vi "HGF_Visitor.appendData2Variant.vi"(0 "initData":variant, 2 "addressee":string, 3 "destination":refnum<class "HGF_TriggeredEvent.lvclass">, 5 "error in (no error)":errorcluster) -> (14 "dup initData":variant, 19 "error out":errorcluster)   [LabVIEW 2014, in "HGF_BaseClasses.lvlib" / "HGF_Visitor.lvclass"]
uses:
  HGF_Visitor.lvclass
  HGF_TriggeredEvent/HGF_TriggeredEvent.lvclass
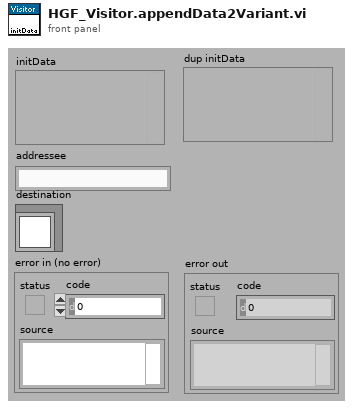
[diagram p1: front panel]
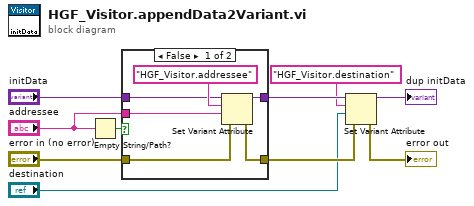
[diagram p0: block diagram]
diagram:
  n1 = Empty String/Path?(string/path="addressee") -> (empty?=w8:bool)
  n2 = case shown="False" w8 {
    tunnel: "addressee" -> [w16 _]
    tunnel: "initData" -> [w14 w18]
    tunnel: [w13 w18] -> w6
    tunnel: "error in (no error)" -> [w12 w17]
    tunnel: [w11 w17] -> w4
    frame False {
      n3 = Set Variant Attribute(Variant=w14, name="HGF_Visitor.addressee", value=w16, error in=w12) -> (Variant out=w13:variant, error out=w11:errorcluster)  [unwired: 1 out]
    }
    frame True {
    }
  }
  n4 = Set Variant Attribute(Variant=w6, name="HGF_Visitor.destination", value="destination", error in=w4) -> (Variant out=→"dup initData":variant, error out=→"error out":errorcluster)  [unwired: 1 out]
